vi "cRIO_v2.vi"() -> ()   [LabVIEW 2015]
uses:
  <vilib>/FPGAPlugInAG/cRIO-9113/niLvFpga_Open_cRIO-9113.vi
  <vilib>/rvi/interface/common/dynamic/niFpgaDynamicAddResources.vi
  <vilib>/Utility/error.llb/Error Cluster From Error Code.vi
  <vilib>/FPGAPlugInAG/Dynamic/niLvFpga_Run_Dynamic.vi
  <vilib>/rvi/interface/common/niFpgaWaitOnOcc.vi
  <vilib>/rvi/errors/niLvFpgaAdjustHostInterfaceError.vi
  <vilib>/FPGAPlugInAG/Dynamic/niLvFpga_Close_Dynamic.vi
  <vilib>/rvi/interface/nirviOpenFPGA/nirviOpenFPGA.xnode
  FPGA Bitfiles/DW40ticks_FPGATarget_Fpgav2_1N2izcJsYEE.lvbitx
  Fpga_v2.vi
  <vilib>/rvi/interface/nirviMethod/nirviMethod.xnode
  <vilib>/rvi/interface/nirviReadWriteControl/nirviReadWriteControl.xnode
  <vilib>/rvi/interface/nirviCloseFPGA/nirviCloseFPGA.xnode
  <vilib>/rvi/errors/niLvFpgaMergeErrorWithErrorCode.vi
  <vilib>/FPGAPlugInAG/Dynamic/niLvFpga_ReadFifo_Dynamic.vi
  <vilib>/rvi/interface/Simulation/niFpgaSimulationCallBeginRW.vi
  <vilib>/FPGAPlugInAG/Dynamic/niLvFpga_StartFifo_Dynamic.vi
  <vilib>/FPGAPlugInAG/Dynamic/niLvFpga_ConfigureFifo_Dynamic.vi
  NiFpgaLv.dll
panel:
  out "error out":errorcluster
  out "Actual Depth of FIFO":u32
  out "Initial write Elements Remaining":u32
  in  "stop":bool
  out "Timed Out?":bool
  out "Number of times timed out":u8
  out "backlog (Elements remaing on the write)":u32
  in  "Data write ON/OFF":bool
  in  "datachanel":bool
  out "Time(ms) for a loop":u32
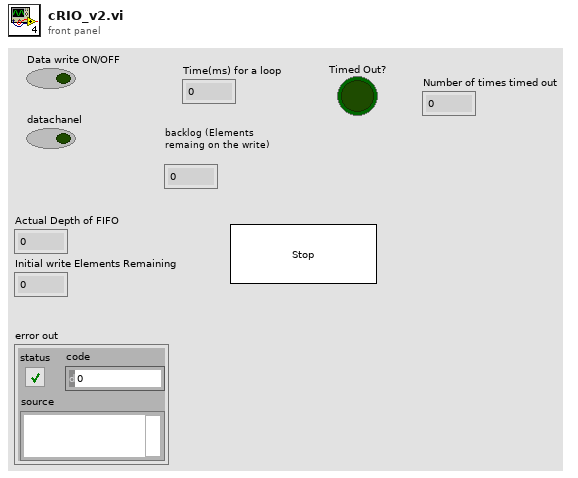
[diagram p1: front panel]
types:
  T1 = enum16{"open", "open or create", "create or replace", "create", "open (read-only)"}
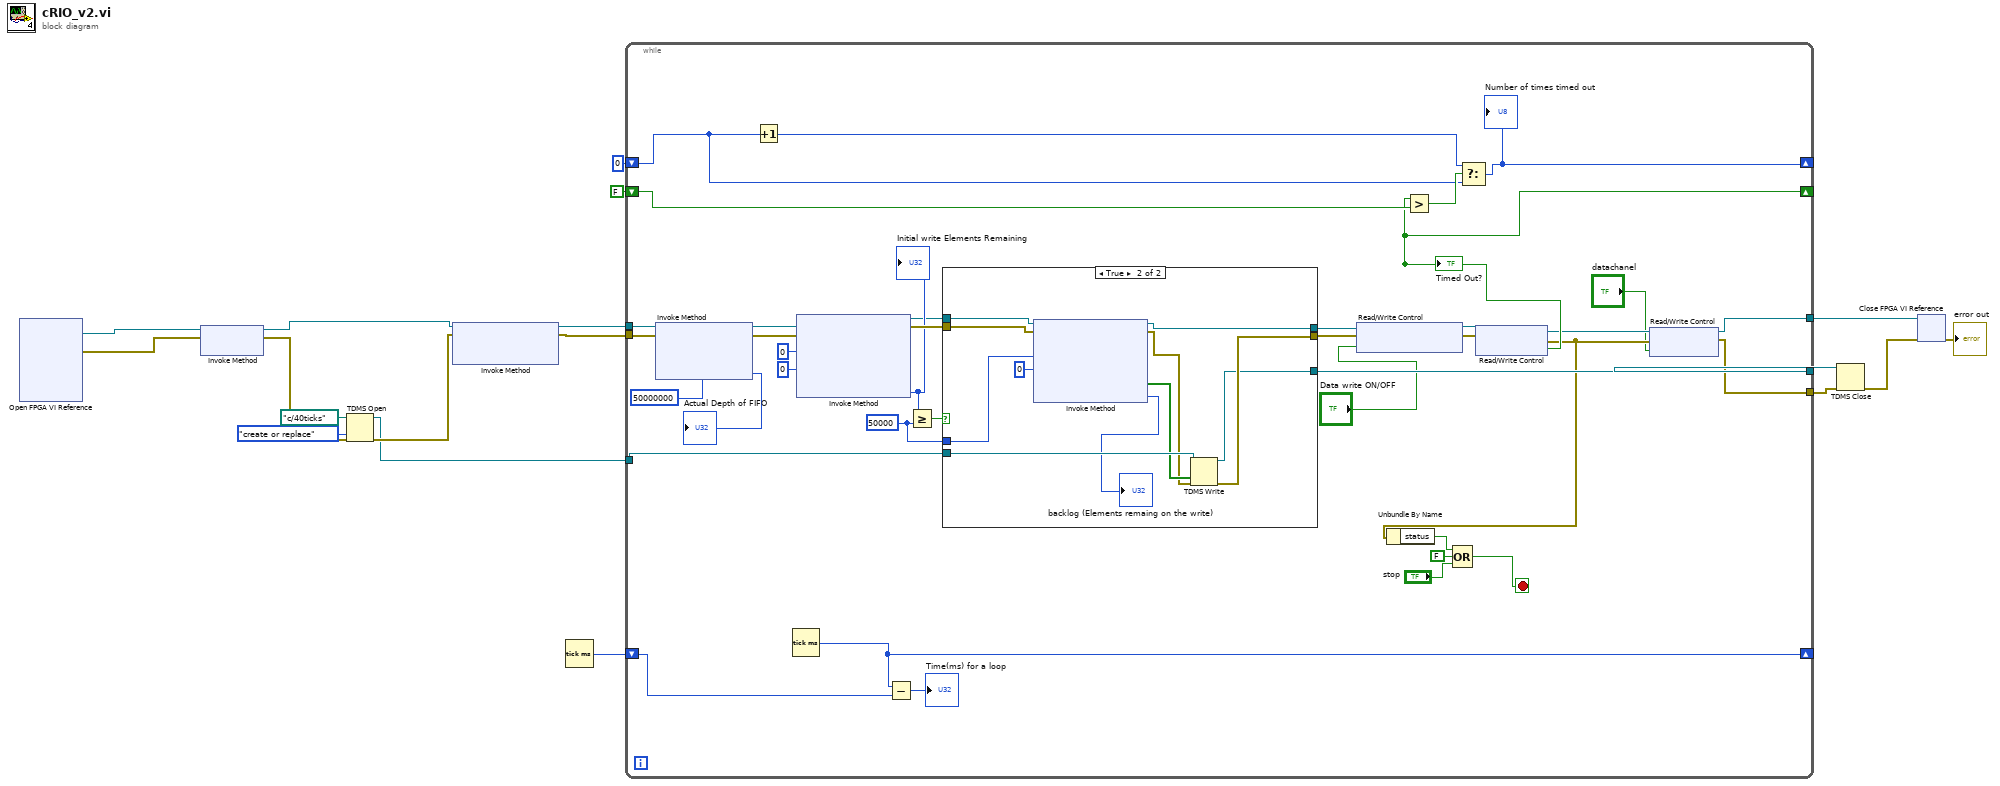
[diagram p0: block diagram]
diagram:
  n1 = xnode "Open FPGA VI Reference"() -> ("FPGA VI Reference Out"=w1:refnum<k20>, "error out"=w2:errorcluster)  [unwired: 2 in]
  n2 = xnode "Invoke Method"("FPGA VI Reference In"=w1, "error in"=w2) -> ("FPGA VI Reference Out"=w17:refnum<k20>, "error out"=w18:errorcluster)
  n3 = TDMS Open(8:w18, 10:T1."create or replace" ("operation (0:open)"), 11:path "c:/40ticks" ("file path")) -> (0:w16:errorcluster, 3:w11:refnum<k34>)  [unwired: 4 in]
  n4 = xnode "Invoke Method"("FPGA VI Reference In"=w17, "error in"=w16) -> ("FPGA VI Reference Out"=w15:refnum<k20>, "error out"=w14:errorcluster)  [unwired: 1 in]
  n5 = Tick Count (ms)() -> (millisecond timer value=w3:u32)
  n6 = while {
    tunnel: w15 -> [w56]
    tunnel: w14 -> [w55]
    tunnel: w11 -> [w47]
    tunnel: [w45] -> w9
    shift-right: [w28] -> _
    shift-left: FALSE ("Timed Out?") -> [w43]
    shift-right: [w39] -> _
    shift-left: u8 0 -> [w41]
    tunnel: [w25] -> w5
    tunnel: [w24] -> w4
    shift-right: [w21] -> _
    shift-left: w3 -> [w22]
    stop <- w44 stop-if-true
    w34 = u32 50000 ("y")
    n7 = xnode "Invoke Method"("FPGA VI Reference In"=w56, "error in"=w55, "Requested Depth"=u32 50000000) -> ("FPGA VI Reference Out"=w52:refnum<k20>, "error out"=w51:errorcluster, "Actual Depth"=→"Actual Depth of FIFO":u32)
    n8 = Increment(x=w41) -> (x+1=w40:u8)
    n9 = Tick Count (ms)() -> (millisecond timer value=w21:u32)
    n10 = xnode "Invoke Method"("FPGA VI Reference In"=w52, "error in"=w51, "Number of Elements"=u32 0, "Timeout (ms)"=0) -> ("FPGA VI Reference Out"=w35:refnum<k20>, "error out"=w48:errorcluster, "Elements Remaining"=w36:u32)  [unwired: 1 out]
    "Initial write Elements Remaining" <- w36
    n11 = Subtract(x=w21, y=w22) -> (x-y=→"Time(ms) for a loop":u32)
    n12 = Greater Or Equal?(x=w36, y=w34) -> (x >= y?=w37:bool)
    n13 = case shown="True" w37 {
      tunnel: w48 -> [w57 w66]
      tunnel: w47 -> [w59 w70]
      tunnel: [w57 w69] -> w32
      tunnel: [w59 w68] -> w45
      tunnel: w35 -> [w58 w67]
      tunnel: [w58 w65] -> w33
      tunnel: w34 -> [_ w62]
      frame False {
      }
      frame True {
        n14 = xnode "Invoke Method"("FPGA VI Reference In"=w67, "error in"=w66, "Number of Elements"=w62, "Timeout (ms)"=0) -> ("FPGA VI Reference Out"=w65:refnum<k20>, "error out"=w63:errorcluster, "Data"=w64:bool[], "Elements Remaining"=→"backlog (Elements remaing on the write)":u32)
        n15 = TDMS Write(0:w70, 9:w64, 11:w63) -> (4:w68:refnum<k34>, 15:w69:errorcluster)  [unwired: 3 in, 2 out]
      }
    }
    n16 = xnode "Read/Write Control"("FPGA VI Reference In"=w33, "error in"=w32, "Data write ON/OFF"="Data write ON/OFF") -> ("FPGA VI Reference Out"=w31:refnum<k20>, "error out"=w30:errorcluster)
    n17 = xnode "Read/Write Control"("FPGA VI Reference In"=w31, "error in"=w30) -> ("FPGA VI Reference Out"=w27:refnum<k20>, "error out"=w26:errorcluster, "Timed Out?"=w28:bool)
    "Timed Out?" <- w28
    n18 = Unbundle By Name(w26) -> ("status"=w38:bool)
    n19 = Greater?(x=w28, y=w43) -> (0:w42:bool)
    n20 = Compound Arithmetic op=OR(w38, FALSE ("value"), "stop") -> (w44:bool)
    n21 = Select(t=w40, s=w42, f=w41) -> (s? t:f=w39:u8)
    "Number of times timed out" <- w39
    n22 = xnode "Read/Write Control"("FPGA VI Reference In"=w27, "error in"=w26, "datachanel"="datachanel") -> ("FPGA VI Reference Out"=w25:refnum<k20>, "error out"=w24:errorcluster)
  }
  n23 = TDMS Close(8:w4, 11:w9) -> (0:w10:errorcluster)  [unwired: 1 out]
  n24 = xnode "Close FPGA VI Reference"("FPGA VI Reference In"=w5, "error in"=w10) -> ("error out"=→"error out":errorcluster)
